vi "Teleop.vi"(10 "Match Info":T1={"Autonomous Elapsed Seconds"=0.0, "TeleOp Elapsed Seconds"=0.0, "Disabled Elapsed Seconds"=0.0, "Visited Autonomous"=FALSE, "Visited TeleOp"=FALSE, "Visited Disabled"=FALSE, "Autonomous Settings"={"Autonomous Style"=enum."Independent", "VI Refnum"=refnum}}, 11 "Call Context":T2) -> ()   [LabVIEW 2011]
doc: "This VI is called for each TeleOp packet received from the DS where the robot is not disabled. It is often used to read from the joysticks and update I/O or to update setpoints for timed control loops. It should complete and return within 20 milliseconds or it may miss DS packets."
uses:
  <vilib>/Rock Robotics/WPI/DriverStation/WPI_DriverStationDerivedRobotMode.ctl
  <vilib>/Rock Robotics/WPI/DriverStation/WPI_DriverStationMatch Info.ctl
  <vilib>/Rock Robotics/WPI/Relay/WPI_RelayValue.ctl
  Robot Global Data.vi
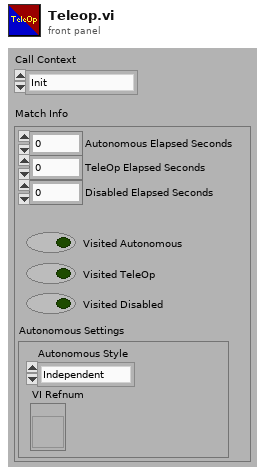
[diagram p1: front panel]
types:
  T1 = typedef "WPI_DriverStationMatch Info.ctl" = cluster{"Autonomous Elapsed Seconds":dbl, "TeleOp Elapsed Seconds":dbl, "Disabled Elapsed Seconds":dbl, "Visited Autonomous":bool, "Visited TeleOp":bool, "Visited Disabled":bool, "Autonomous Settings":cluster{"Autonomous Style":enum16{"Iterative", "Independent"}, "VI Refnum":refnum<vi>}}
  T2 = typedef "WPI_DriverStationDerivedRobotMode.ctl" = enum16{"Init", "Execute", "Stop"}
  T3 = typedef "WPI_RelayValue.ctl" = enum16{"Off", "On", "Forward", "Reverse"}
  T4 = typedef "WPI_JoystickDevRef.ctl" = cluster{"Device":T5}
  T5 = typedef "WPI_JoystickDeviceEnum.ctl" = enum16{"USB 1", "USB 2", "USB 3", "USB 4", "Kinect 1", "Kinect 2"}
  T6 = typedef "WPI_JoystickButtonState.ctl" = cluster{"Button 1":bool, "Button 2":bool, "Button 3":bool, "Button 4":bool, "Button 5":bool, "Button 6":bool, "Button 7":bool, "Button 8":bool, "Button 9":bool, "Button 10":bool, "Button 11":bool, "Button 12":bool}
  T7 = cluster{"axis 1 (x)":dbl, "axis 2 (y)":dbl, "axis 3 (throttle)":dbl, "axis 4":dbl, "axis 5":dbl, "axis 6":dbl}
  T8 = typedef "WPI_MotorControlDeviceRef.ctl" = cluster{"DeviceStatus":errorcluster, "Type":enum16{"PWM", "CAN"}, "PWM":cluster{"Digital Module":T9, "PWM Channel":T10, "DeadBand":T11}, "CAN":cluster{"Device Number":u8, "Control Mode":T12, "Semaphore":T13, "Max Vout":dbl}, "Invert":bool, "TransformRef":T14, "InvTransformRef":T14}
  T9 = typedef "FPGA_TypedefDigitalModule.ctl" = enum16{"Digital Module 1", "Digital Module 2"}
  T10 = typedef "FPGA_DIOPWMChannel.ctl" = enum8{"PWM 1", "PWM 2", "PWM 3", "PWM 4", "PWM 5", "PWM 6", "PWM 7", "PWM 8", "PWM 9", "PWM 10", "Invalid"}
  T11 = typedef "WPI_PWMDeadband.ctl" = cluster{"Name":string, "maxPositivePwm":i32, "minPositivePwm":i32, "centerPwm":i32, "maxNegativePwm":i32, "minNegativePwm":i32, "angularRange":u16}
  T12 = typedef "WPI_CANJaguar_ControlMode.ctl" = enum8{"Percent VBus", "Current", "Speed", "Position", "Voltage"}
  T13 = typedef "Semaphore RefNum" = refnum<k1>
  T14 = typedef "WPI_PWMTransform_ConPane.ctl" = refnum<vi>
  T15 = cluster{"Driver Station Digital Input (1-8)[0]":bool, "Driver Station Digital Input (1-8)[1]":bool, "Driver Station Digital Input (1-8)[2]":bool, "Driver Station Digital Input (1-8)[3]":bool, "Driver Station Digital Input (1-8)[4]":bool, "Driver Station Digital Input (1-8)[5]":bool, "Driver Station Digital Input (1-8)[6]":bool, "Driver Station Digital Input (1-8)[7]":bool, "Driver Station Digital Input (1-8)[8]":bool}
  T16 = typedef "WPI_RelayDevRef.ctl" = cluster{"DevStatus":errorcluster, "Relay Channel":T17, "Digital Module":T9, "Relay Direction":T18}
  T17 = typedef "FPGA_DIORelayChannel.ctl" = enum8{"Relay 1", "Relay 2", "Relay 3", "Relay 4", "Relay 5", "Relay 6", "Relay 7", "Relay 8", "Invalid"}
  T18 = typedef "WPI_RelayDirection.ctl" = enum16{"Both directions", "Forward only", "Reverse only"}
  T19 = typedef "WPI_DigitalInputDevRef.ctl" = cluster{"DevStatus":errorcluster, "DIO Channel":T20, "Digital Module":T9}
  T20 = typedef "FPGA_DIOChannel.ctl" = enum8{"DIO 1", "DIO 2", "DIO 3", "DIO 4", "DIO 5", "DIO 6", "DIO 7", "DIO 8", "DIO 9", "DIO 10", "DIO 11", "DIO 12", "DIO 13", "DIO 14", "Invalid"}
  T21 = typedef "WPI_ServoDeviceRef.ctl" = cluster{"DeviceStatus":errorcluster, "Digital Module":T9, "PWM Channel":T10, "DeadBand":T11}
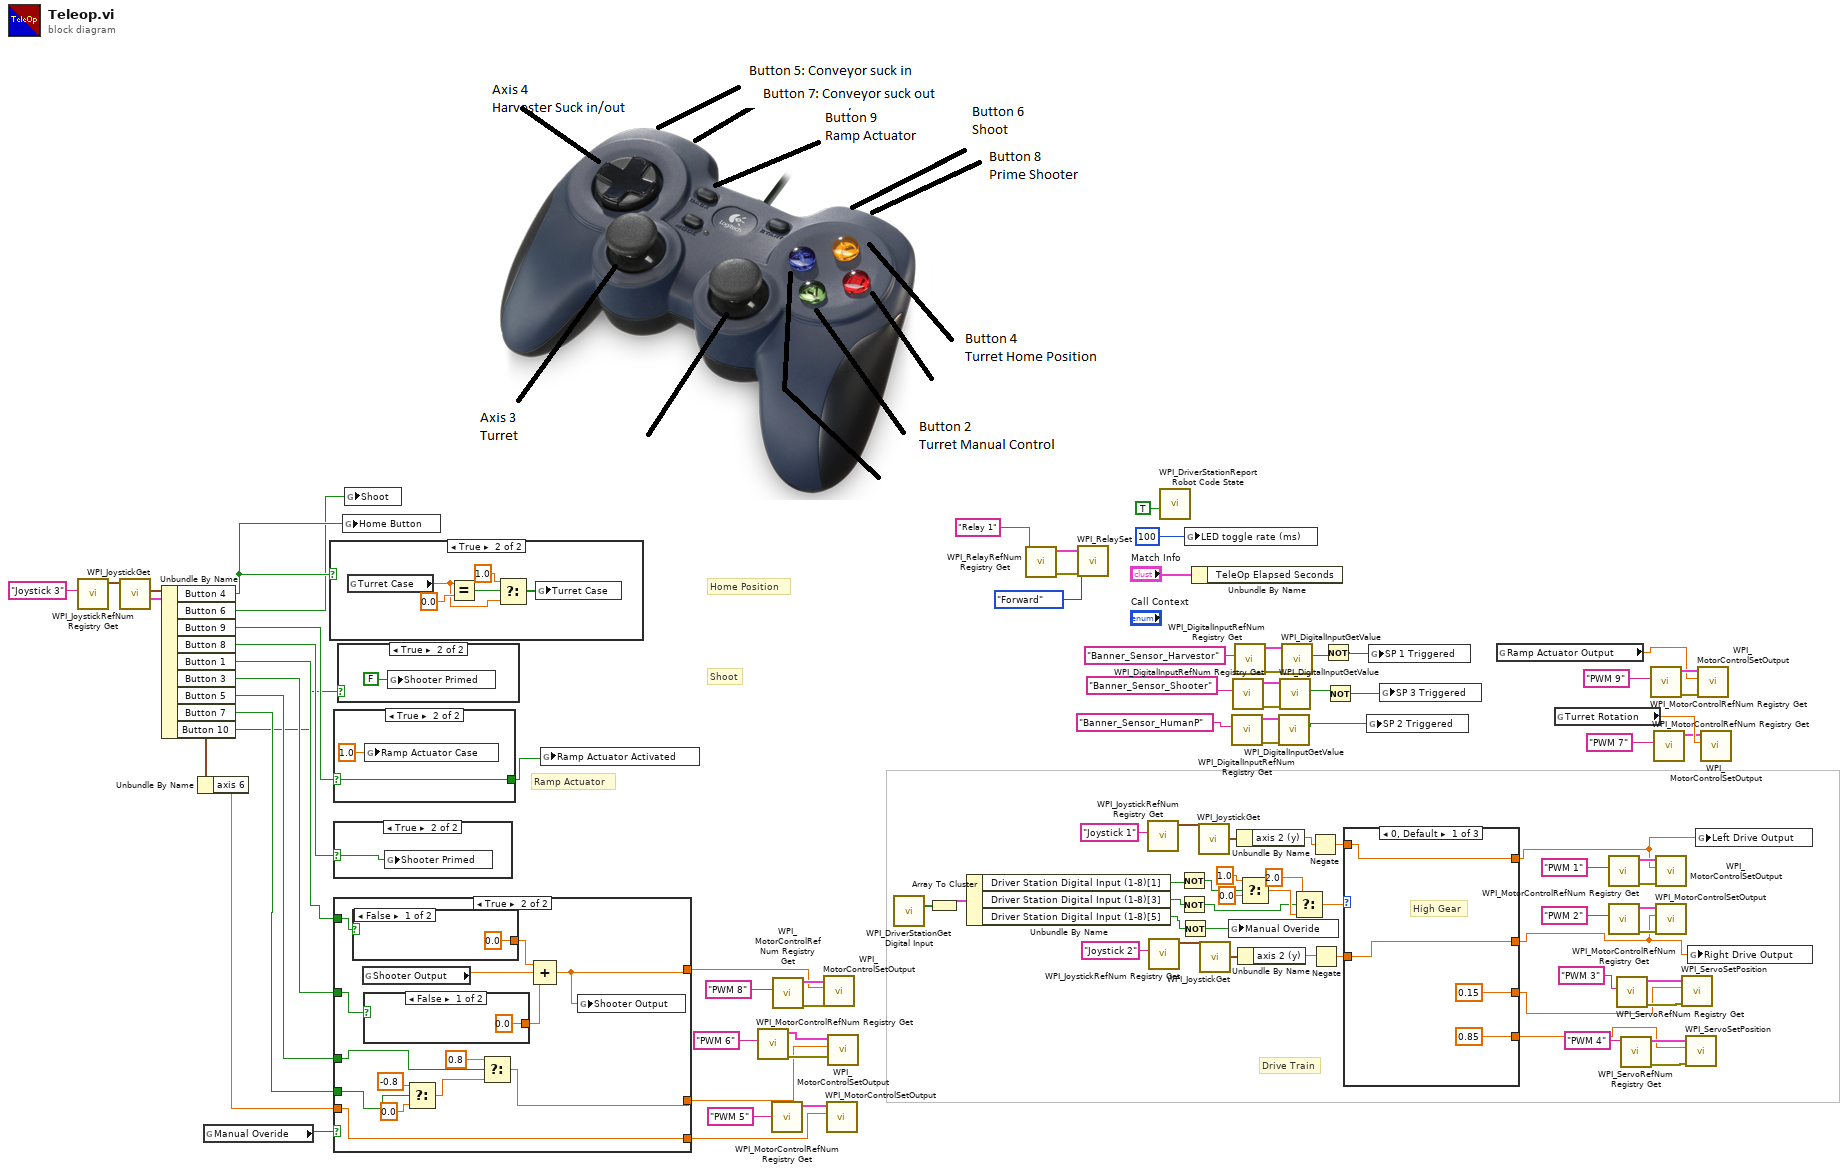
[diagram p0: block diagram]
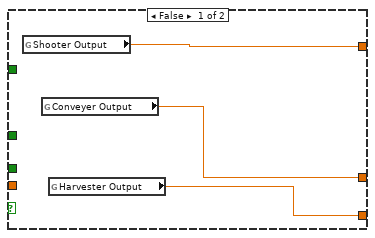
[diagram p3: hidden frame]
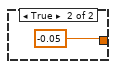
[diagram p4: hidden frame]
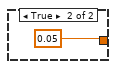
[diagram p5: hidden frame]
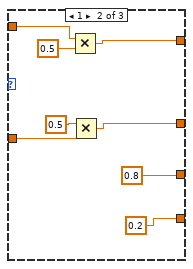
[diagram p9: hidden frame]
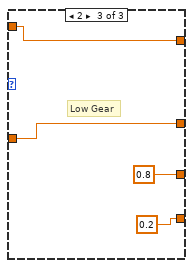
[diagram p10: hidden frame]
diagram:
  # "Home Position"
  # "Shoot"
  # "Ramp Actuator"
  # "Drive Train"
  n1 = call <vilib>:"WPI_JoystickRefNum Registry Get.vi"("refnum name"="Joystick 3") -> ("JoystickDevRef"=w46:T4)  [unwired: 9 in, 1 out]
  n2 = call <vilib>:"WPI_JoystickGet.vi"("JoystickDevRef"=w46) -> ("Buttons"=w47:T6, "Axes"=w18:T7)  [unwired: 4 in, 1 out]
  n3 = Unbundle By Name(w47) -> ("Button 4"=w45:bool, "Button 6"=w44:bool, "Button 9"=w43:bool, "Button 8"=w19:bool, "Button 1"=w13:bool, "Button 3"=w12:bool, "Button 5"=w11:bool, "Button 7"=w10:bool, "Button 10"=w1:bool)
  n4 = Unbundle By Name(w18) -> ("axis 6"=w5:dbl)
  n5 = global read "Robot Global Data.vi" "Manual Overide"() -> (w4:bool)
  n6 = case shown="True" w45 {
    frame False {
    }
    frame True {
      n7 = global read "Robot Global Data.vi" "Turret Case"() -> (w96:dbl)
      n8 = Equal?(x=w96, y=0.0) -> (x = y?=w98:bool)
      n9 = Select(t=1.0, s=w98, f=w96) -> (s? t:f=w95:dbl)
      n10 = global write "Robot Global Data.vi" "Turret Case"(w95) -> ()
    }
  }
  n11 = case shown="True" w43 {
    selector: w43 -> [w100 w102]
    tunnel: [w100 w102] -> w49
    frame False {
    }
    frame True {
      n12 = global write "Robot Global Data.vi" "Ramp Actuator Case"(1.0 ("Ramp Actuator Case")) -> ()
    }
  }
  n13 = case shown="True" w19 {
    selector: w19 -> [_ w103]
    frame False {
    }
    frame True {
      n14 = global write "Robot Global Data.vi" "Shooter Primed"(w103) -> ()
    }
  }
  n15 = case shown="True" w4 {
    tunnel: [w106 w107] -> w14
    tunnel: w13 -> [_ w112]
    tunnel: w12 -> [_ w111]
    tunnel: w11 -> [_ w115]
    tunnel: w10 -> [_ w116]
    tunnel: [w104 w114] -> w6
    tunnel: w5 -> [_ w113]
    tunnel: [w105 w113] -> w3
    frame False {
      n16 = global read "Robot Global Data.vi" "Shooter Output"() -> (w106:dbl)
      n17 = global read "Robot Global Data.vi" "Conveyer Output"() -> (w104:dbl)
      n18 = global read "Robot Global Data.vi" "Harvester Output"() -> (w105:dbl)
    }
    frame True {
      n19 = case shown="False" w112 {
        tunnel: [0.0 0.05] -> w110
        frame False {
        }
        frame True {
        }
      }
      n20 = global read "Robot Global Data.vi" "Shooter Output"() -> (w108:dbl)
      n21 = case shown="False" w111 {
        tunnel: [0.0 -0.05] -> w109
        frame False {
        }
        frame True {
        }
      }
      n22 = Select(t=-0.8, s=w116, f=0.0) -> (s? t:f=w120:dbl)
      n23 = Select(t=0.8, s=w115, f=w120) -> (s? t:f=w114:dbl)
      n24 = Compound Arithmetic op=ADD(w110, w108, w109) -> (w107:dbl)
      n25 = global write "Robot Global Data.vi" "Shooter Output"(w107) -> ()
    }
  }
  n26 = case shown="True" w1 {
    frame False {
    }
    frame True {
      n27 = global write "Robot Global Data.vi" "Shooter Primed"(FALSE ("Shooter Primed")) -> ()
    }
  }
  n28 = global write "Robot Global Data.vi" "Home Button"(w45) -> ()
  n29 = global write "Robot Global Data.vi" "Shoot"(w44) -> ()
  n30 = global write "Robot Global Data.vi" "Ramp Actuator Activated"(w49) -> ()
  n31 = call <vilib>:"WPI_MotorControlRefNum Registry Get.vi"("refnum name"="PWM 6") -> ("error out"=w7:errorcluster, "MotorControlDevRef"=w8:T8)  [unwired: 9 in]
  n32 = call <vilib>:"WPI_MotorControlRefNum Registry Get.vi"("refnum name"="PWM 5") -> ("MotorControlDevRef"=w37:T8)  [unwired: 9 in, 1 out]
  n33 = call <vilib>:"WPI_MotorControlRefNum Registry Get.vi"("refnum name"="PWM 8") -> ("error out"=w21:errorcluster, "MotorControlDevRef"=w22:T8)  [unwired: 9 in]
  n34 = call <vilib>:"WPI_MotorControlSetOutput.vi"("error in (no error)"=w21, "Output"=w14, "MotorControlDevRef"=w22) -> ()  [unwired: 7 in, 2 out]
  n35 = call <vilib>:"WPI_MotorControlSetOutput.vi"("Output"=w3, "MotorControlDevRef"=w37) -> ()  [unwired: 8 in, 2 out]
  n36 = call <vilib>:"WPI_MotorControlSetOutput.vi"("error in (no error)"=w7, "Output"=w6, "MotorControlDevRef"=w8) -> ()  [unwired: 7 in, 2 out]
  n37 = call <vilib>:"WPI_DriverStationGet Digital Input.vi"() -> ("Driver Station Digital Input (1-8)"=w68:bool[])  [unwired: 11 in]
  n38 = Array To Cluster(array=w68) -> (cluster=w91:T15)
  n39 = Unbundle By Name(w91) -> ("Driver Station Digital Input (1-8)[1]"=w71:bool, "Driver Station Digital Input (1-8)[3]"=w70:bool, "Driver Station Digital Input (1-8)[5]"=w15:bool)
  n40 = call <vilib>:"WPI_RelayRefNum Registry Get.vi"("refnum name"="Relay 1") -> ("error out"=w41:errorcluster, "RelayDevRef"=w42:T16)  [unwired: 9 in]
  n41 = call <vilib>:"WPI_RelaySet.vi"("error in (no error)"=w41, "RelayValue"=WPI_RelayValue."Forward", "RelayDevRef"=w42) -> ()  [unwired: 7 in, 2 out]
  n42 = call <vilib>:"WPI_JoystickRefNum Registry Get.vi"("refnum name"="Joystick 1") -> ("JoystickDevRef"=w84:T4)  [unwired: 9 in, 1 out]
  n43 = call <vilib>:"WPI_JoystickRefNum Registry Get.vi"("refnum name"="Joystick 2") -> ("JoystickDevRef"=w81:T4)  [unwired: 9 in, 1 out]
  n44 = call <vilib>:"WPI_DriverStationReport Robot Code State.vi"("TeleOp"=TRUE ("Autonomous")) -> ()  [unwired: 10 in, 1 out]
  n45 = Not(x=w71) -> (.not. x?=w69:bool)
  n46 = Not(x=w70) -> (.not. x?=w17:bool)
  n47 = Not(x=w15) -> (.not. x?=w16:bool)
  n48 = global write "Robot Global Data.vi" "LED toggle rate (ms)"(u32 100 ("LED ms toggle rate")) -> ()
  n49 = Unbundle By Name("Match Info") -> ()  [unwired: 1 out]
  n50 = call <vilib>:"WPI_JoystickGet.vi"("JoystickDevRef"=w84) -> ("Axes"=w83:T7)  [unwired: 4 in, 2 out]
  n51 = call <vilib>:"WPI_JoystickGet.vi"("JoystickDevRef"=w81) -> ("Axes"=w82:T7)  [unwired: 4 in, 2 out]
  n52 = global write "Robot Global Data.vi" "Manual Overide"(w16) -> ()
  n53 = call <vilib>:"WPI_DigitalInputRefNum Registry Get.vi"("refnum name"="Banner_Sensor_HumanP") -> ("error out"=w32:errorcluster, "DigitalInputDevRef"=w31:T19)  [unwired: 9 in]
  n54 = call <vilib>:"WPI_DigitalInputRefNum Registry Get.vi"("refnum name"="Banner_Sensor_Shooter") -> ("error out"=w33:errorcluster, "DigitalInputDevRef"=w34:T19)  [unwired: 9 in]
  n55 = call <vilib>:"WPI_DigitalInputRefNum Registry Get.vi"("refnum name"="Banner_Sensor_Harvestor") -> ("error out"=w36:errorcluster, "DigitalInputDevRef"=w35:T19)  [unwired: 9 in]
  n56 = Unbundle By Name(w83) -> ("axis 2 (y)"=w67:dbl)
  n57 = Unbundle By Name(w82) -> ("axis 2 (y)"=w65:dbl)
  n58 = Select(t=1.0, s=w69, f=0.0 ("t")) -> (s? t:f=w88:dbl)
  n59 = call <vilib>:"WPI_DigitalInputGetValue.vi"("error in (no error)"=w32, "DigitalInputDevRef"=w31) -> ("Value"=w27:bool)  [unwired: 7 in, 2 out]
  n60 = call <vilib>:"WPI_DigitalInputGetValue.vi"("error in (no error)"=w33, "DigitalInputDevRef"=w34) -> ("Value"=w26:bool)  [unwired: 7 in, 2 out]
  n61 = call <vilib>:"WPI_DigitalInputGetValue.vi"("error in (no error)"=w36, "DigitalInputDevRef"=w35) -> ("Value"=w24:bool)  [unwired: 7 in, 2 out]
  n62 = Select(t=2.0, s=w17, f=w88) -> (s? t:f=w86:dbl)
  n63 = Negate(x=w67) -> (-x=w66:dbl)
  n64 = Negate(x=w65) -> (-x=w64:dbl)
  n65 = Not(x=w24) -> (.not. x?=w23:bool)
  n66 = Not(x=w26) -> (.not. x?=w25:bool)
  n67 = case shown="0, Default" w86 {
    tunnel: w64 -> [w129 w134 w141]
    tunnel: [w129 w135 w141] -> w56
    tunnel: [w128 w136 w140] -> w57
    tunnel: [0.15 ("LeftShifter_Pos") 0.8 0.8] -> w73
    tunnel: [0.85 0.2 ("LeftShifter_Pos") 0.2 ("LeftShifter_Pos")] -> w72
    tunnel: w66 -> [w128 w132 w140]
    frame 0, Default {
      # "High Gear"
    }
    frame 1 {
      n68 = Multiply(x=w132, y=0.5) -> (x*y=w136:dbl)
      n69 = Multiply(x=0.5 ("y"), y=w134) -> (x*y=w135:dbl)
    }
    frame 2 {
      # "Low Gear"
    }
  }
  n70 = global write "Robot Global Data.vi" "SP 2 Triggered"(w27) -> ()
  n71 = global write "Robot Global Data.vi" "SP 1 Triggered"(w23) -> ()
  n72 = global write "Robot Global Data.vi" "SP 3 Triggered"(w25) -> ()
  n73 = global read "Robot Global Data.vi" "Ramp Actuator Output"() -> (w2:dbl)
  n74 = global read "Robot Global Data.vi" "Turret Rotation"() -> (w52:dbl)
  n75 = call <vilib>:"WPI_MotorControlRefNum Registry Get.vi"("refnum name"="PWM 1") -> ("error out"=w61:errorcluster, "MotorControlDevRef"=w63:T8)  [unwired: 9 in]
  n76 = call <vilib>:"WPI_MotorControlRefNum Registry Get.vi"("refnum name"="PWM 2") -> ("error out"=w60:errorcluster, "MotorControlDevRef"=w59:T8)  [unwired: 9 in]
  n77 = call <vilib>:"WPI_ServoRefNum Registry Get.vi"("refnum name"="PWM 3") -> ("error out"=w77:errorcluster, "ServoDeviceRef"=w78:T21)  [unwired: 9 in]
  n78 = call <vilib>:"WPI_ServoRefNum Registry Get.vi"("refnum name"="PWM 4") -> ("error out"=w76:errorcluster, "ServoDeviceRef"=w75:T21)  [unwired: 9 in]
  n79 = call <vilib>:"WPI_MotorControlRefNum Registry Get.vi"("refnum name"="PWM 9") -> ("error out"=w54:errorcluster, "MotorControlDevRef"=w53:T8)  [unwired: 9 in]
  n80 = call <vilib>:"WPI_MotorControlRefNum Registry Get.vi"("refnum name"="PWM 7") -> ("MotorControlDevRef"=w50:T8)  [unwired: 9 in, 1 out]
  n81 = call <vilib>:"WPI_MotorControlSetOutput.vi"("error in (no error)"=w61, "Output"=w57, "MotorControlDevRef"=w63) -> ()  [unwired: 7 in, 2 out]
  n82 = call <vilib>:"WPI_MotorControlSetOutput.vi"("error in (no error)"=w60, "Output"=w56, "MotorControlDevRef"=w59) -> ()  [unwired: 7 in, 2 out]
  n83 = call <vilib>:"WPI_ServoSetPosition.vi"("error in (no error)"=w77, "Position"=w73, "ServoDeviceRef"=w78) -> ()  [unwired: 7 in, 2 out]
  n84 = call <vilib>:"WPI_ServoSetPosition.vi"("error in (no error)"=w76, "Position"=w72, "ServoDeviceRef"=w75) -> ()  [unwired: 7 in, 2 out]
  n85 = global write "Robot Global Data.vi" "Right Drive Output"(w56) -> ()
  n86 = global write "Robot Global Data.vi" "Left Drive Output"(w57) -> ()
  n87 = call <vilib>:"WPI_MotorControlSetOutput.vi"("error in (no error)"=w54, "Output"=w2, "MotorControlDevRef"=w53) -> ()  [unwired: 7 in, 2 out]
  n88 = call <vilib>:"WPI_MotorControlSetOutput.vi"("Output"=w52, "MotorControlDevRef"=w50) -> ()  [unwired: 8 in, 2 out]
